vi "MotorMultiOff.vi"(3 "Motors":string[](array[string]), 9 "error in (no error)":errorcluster) -> (6 "error out":errorcluster)   [LabVIEW 2009]
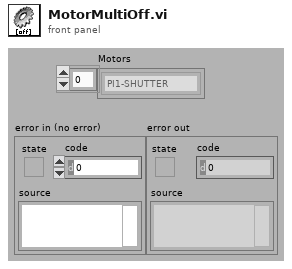
[diagram p1: front panel]
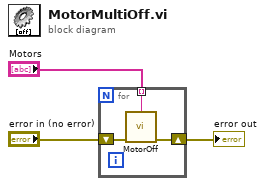
[diagram p0: block diagram]
diagram:
  n1 = for {
    tunnel: "Motors" -> [w4] mode=indexing
    shift-right: [w5] -> w2
    shift-left: "error in (no error)" -> [w6]
    n2 = call "MotorOff.vi"(2:w4, "error in (no error)"=w6) -> ("error out"=w5:errorcluster)  [unwired: 6 in, 1 out]
  }
  "error out" <- w2
